vi "ni579x Configure LO Enable.vi"(0 "Register Bus":refnum<class "ni579x Register Bus v1 Host.lvclass">=refnum, 1 "scope":string(combo)="LO1", 5 "enable?":bool=TRUE, 7 "wait for enable completion?":bool=TRUE, 11 "Error In":errorcluster) -> (4 "Register Bus (out)":refnum<class "ni579x Register Bus v1 Host.lvclass">, 15 "Error Out":errorcluster)   [LabVIEW 2013]
uses:
  <instrlib>/ni579x/Register Bus/v1/Host/ni579x Register Bus v1 Host.lvclass
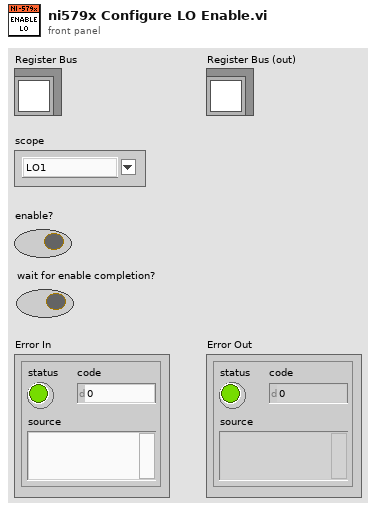
[diagram p1: front panel]
types:
  T1 = typedef "ni579x User Command.ctl" = cluster{"User Data 0":u8, "User Data 1":u8, "User Command ID":T2}
  T2 = typedef "ni579x User Command ID.ctl" = u8
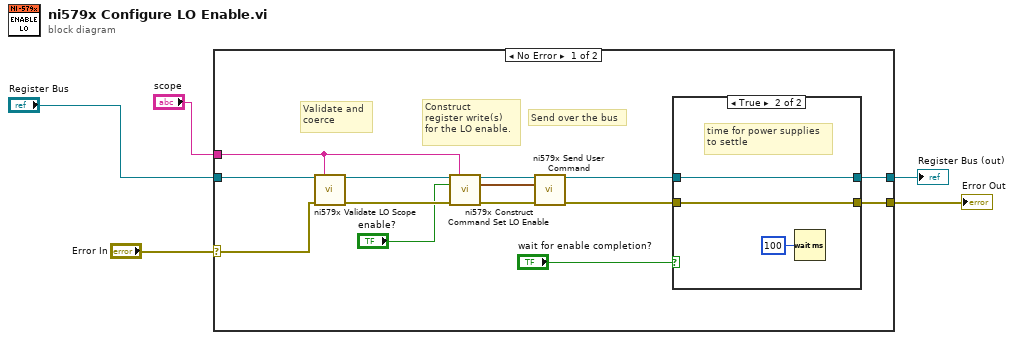
[diagram p0: block diagram]
diagram:
  n1 = case shown="No Error" "Error In" {
    selector: "Error In" -> [w18 w26]
    tunnel: [w6 w26] -> w4
    tunnel: "Register Bus" -> [w19 w25]
    tunnel: [w7 w25] -> w2
    tunnel: "scope" -> [w15 _]
    frame No Error {
      # "Construct\nregister write(s)\nfor the LO enable."
      # "Send over the bus"
      # "Validate and \ncoerce"
      n2 = call <instrlib>:"ni579x Validate LO Scope.vi"("Register Bus"=w19, "scope"=w15, "Error In"=w18) -> ("Register Bus (out)"=w17:refnum<class "ni579x Register Bus v1 Host.lvclass">, "Error Out"=w16:errorcluster)  [unwired: 11 in]
      n3 = call <instrlib>:"ni579x Construct Command Set LO Enable.vi"("Register Bus"=w17, "scope"=w15, "enable?"="enable?", "Error In"=w16) -> ("Register Bus (out)"=w14:refnum<class "ni579x Register Bus v1 Host.lvclass">, "User Command"=w13:T1, "Error Out"=w12:errorcluster)  [unwired: 9 in]
      n4 = call <instrlib>:"ni579x Send User Command.vi"("Register Bus"=w14, "User Command"=w13, "Error In"=w12) -> ("Register Bus (out)"=w9:refnum<class "ni579x Register Bus v1 Host.lvclass">, "Error Out"=w8:errorcluster)  [unwired: 8 in, 3 out]
      n5 = case shown="True" "wait for enable completion?" {
        tunnel: w9 -> [w21 w23]
        tunnel: w8 -> [w20 w22]
        tunnel: [w21 w23] -> w7
        tunnel: [w20 w22] -> w6
        frame False {
        }
        frame True {
          # "time for power supplies\nto settle"
          n6 = Wait (ms)(milliseconds to wait=u32 100) -> ()  [unwired: 1 out]
        }
      }
    }
    frame Error {
    }
  }
  "Register Bus (out)" <- w2
  "Error Out" <- w4
